vi "friction comp.vi"(6 "Vneg":dbl, 7 "Cneg":dbl, 9 "Cpos":dbl, 10 "output y(t)":dbl, 11 "Vpos":dbl) -> (3 "2":dbl)   [LabVIEW 2021]
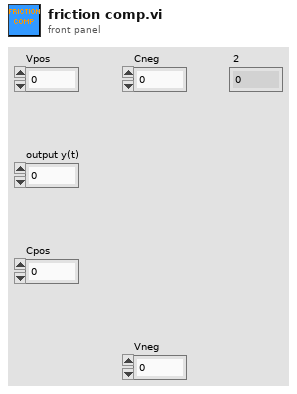
[diagram p1: front panel]
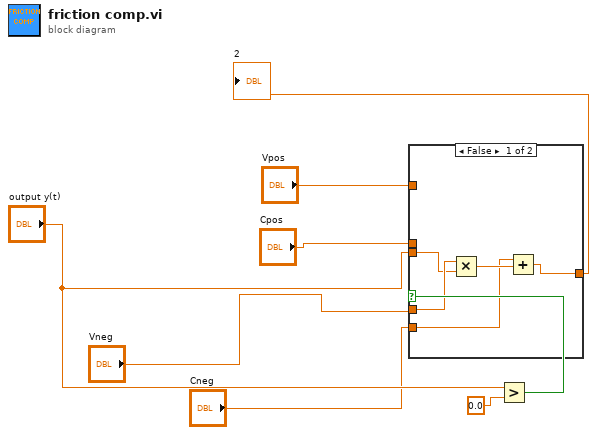
[diagram p0: block diagram]
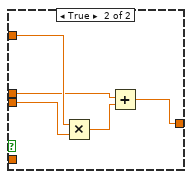
[diagram p2: hidden frame]
diagram:
  n1 = Greater?(x="output y(t)", y=0.0) -> (0:w8:bool)
  n2 = case shown="False" w8 {
    tunnel: [w11 w17] -> w1
    tunnel: "Vneg" -> [w13 _]
    tunnel: "Cneg" -> [w9 _]
    tunnel: "output y(t)" -> [w12 w16]
    tunnel: "Vpos" -> [_ w15]
    tunnel: "Cpos" -> [_ w14]
    frame False {
      n3 = Multiply(x=w13, y=w12) -> (x*y=w10:dbl)
      n4 = Add(x=w9, y=w10) -> (x+y=w11:dbl)
    }
    frame True {
      n5 = Multiply(x=w15, y=w16) -> (x*y=w18:dbl)
      n6 = Add(x=w14, y=w18) -> (x+y=w17:dbl)
    }
  }
  "2" <- w1
